vi "Add Item to the Cabinet.vi"(8 "Object":refnum<class "XRay Scene.lvclass">, 11 "XRay Cabinet In":refnum<class "XRay Cabinet.lvclass">) -> (3 "XRay Cabinet Out":refnum<class "XRay Cabinet.lvclass">)   [LabVIEW 2026, in "XRay Cabinet.lvclass"]
uses:
  XRay Cabinet.lvclass
  XRay Scene/XRay Scene.lvclass
  XRay Cabinet.lvclass/XRay Cabinet.ctl
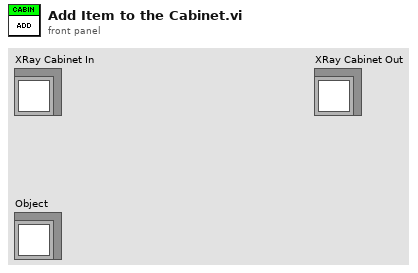
[diagram p1: front panel]
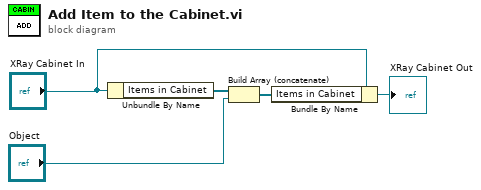
[diagram p0: block diagram]
diagram:
  n1 = Unbundle By Name("XRay Cabinet In") -> ("Items in Cabinet"=w3:refnum<class "XRay Scene.lvclass">[])
  n2 = Build Array (concatenate)(w3, "Object") -> (w1:refnum<class "XRay Scene.lvclass">[])
  n3 = Bundle By Name(cluster="XRay Cabinet In", "Items in Cabinet"=w1) -> (→"XRay Cabinet Out":refnum<class "XRay Cabinet.lvclass">)
